vi "CalculateErrorInLeftPosition__slk_mt.vi"(3 "add error configure":T2, 7 "position in":T1, 8 "error in (no error)":errorcluster, 11 "origin (0,0)":T3) -> (0 "error out":errorcluster, 5 "position out":T1)   [LabVIEW 2012, in "Lazyboots Menu Tool.lvlib"]
doc: "Gets error in left position."
uses:
  Library/Lazyboots Menu Tool.lvlib
  <vilib>/Utility/miscctls.llb/LVPointTypeDef.ctl
  TypeDef/TypeDef_AddErrorConfigure__slk_mt.ctl
  <vilib>/Utility/miscctls.llb/LVPositionTypeDef.ctl
panel:
  # "CalculateErrorInLeftPosition__slk_mt.vi\nGets error in left position.\n\nNOTICE -- YOU MUST LEAVE THIS NOTICE IN PLACE.\n\nCopyright (c) 2011, LIANG LIU Shawn.Liu.cn@gmail.com\nAll rights reserved.\n\nRedistribution and use in source and binary forms, with or without modification, are permitted provided that the following conditions are met:\n-Redistributions of source code must retain the above copyright notice, this list of conditions and the following disclaimer.\n-Redistributions in binary form must reproduce the above copyright notice, this list of conditions and the following disclaimer in the documentation and/or other materials provided with the distribution.\n-Neither the name of the eLp nor the names of its contributors may be used to endorse or promote products derived from this software without specific prior written permission.\n\nTHIS SOFTWARE IS PROVIDED BY THE COPYRIGHT HOLDERS AND CONTRIBUTORS \"AS IS\" AND ANY EXPRESS OR IMPLIED WARRANTIES, INCLUDING, BUT NOT LIMITED TO, THE IMPLIED WARRANTIES OF MERCHANTABILITY AND FITNESS FOR A PARTICULAR PURPOSE ARE DISCLAIMED. IN NO EVENT SHALL THE COPYRIGHT HOLDER OR CONTRIBUTORS BE LIABLE FOR ANY DIRECT, INDIRECT, INCIDENTAL, SPECIAL, EXEMPLARY, OR CONSEQUENTIAL DAMAGES (INCLUDING, BUT NOT LIMITED TO, PROCUREMENT OF SUBSTITUTE GOODS OR SERVICES; LOSS OF USE, DATA, OR PROFITS; OR BUSINESS INTERRUPTION) HOWEVER CAUSED AND ON ANY THEORY OF LIABILITY, WHETHER IN CONTRACT, STRICT LIABILITY, OR TORT (INCLUDING NEGLIGENCE OR OTHERWISE) ARISING IN ANY WAY OUT OF THE USE OF THIS SOFTWARE, EVEN IF ADVISED OF THE POSSIBILITY OF SUCH DAMAGE."
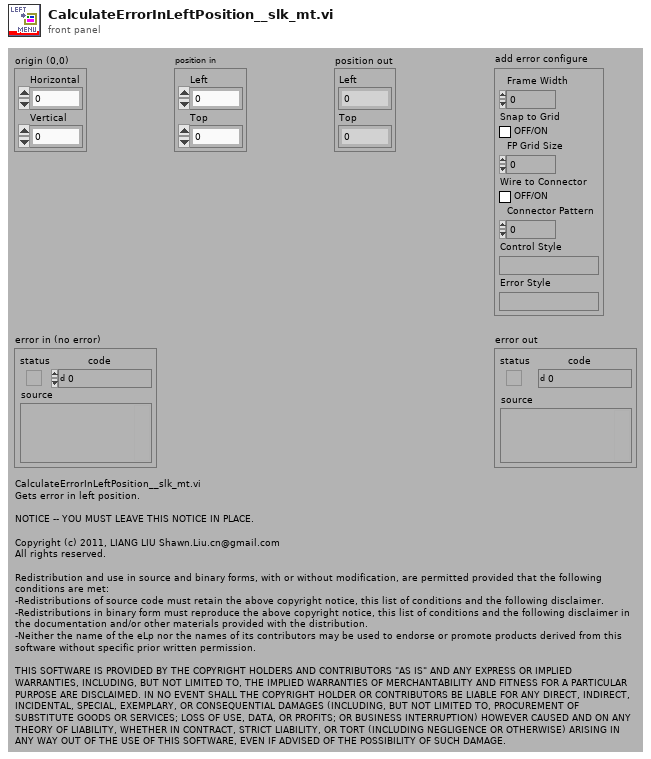
[diagram p1: front panel]
types:
  T1 = typedef "LVPositionTypeDef.ctl" = cluster{"Left":i32, "Top":i32}
  T2 = typedef "Lazyboots Menu Tool.lvlib/TypeDef_AddErrorConfigure__slk_mt.ctl" = cluster{"Frame Width":u32, "Snap to Grid":bool, "FP Grid Size":u32, "Wire to Connector":bool, "Connector Pattern":u32, "Control Style":string, "Error Style":string}
  T3 = typedef "LVPointTypeDef.ctl" = cluster{"Horizontal":i16, "Vertical":i16}
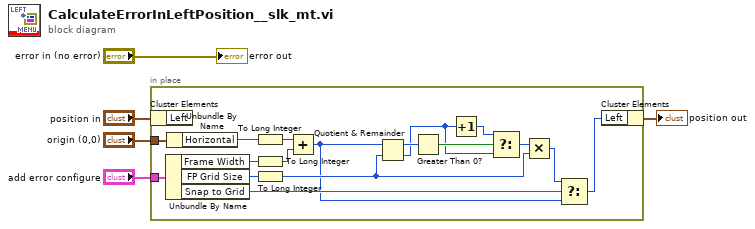
[diagram p0: block diagram]
diagram:
  n1 = in-place {
    in-place-border: "add error configure" -> [w12]
    in-place-border: "origin (0,0)" -> [w9]
    n2 = in-place-cluster #1("position in") -> ()  [unwired: 1 out]
    n3 = Unbundle By Name(w12) -> ("Frame Width"=w22:u32, "FP Grid Size"=w19:u32, "Snap to Grid"=w10:bool)
    n4 = Unbundle By Name(w9) -> ("Horizontal"=w21:i16)
    n5 = To Long Integer(number=w21) -> (32bit integer=w7:i32)
    n6 = To Long Integer(number=w22) -> (32bit integer=w20:i32)
    n7 = To Long Integer(number=w19) -> (32bit integer=w13:i32)
    n8 = Add(x=w7, y=w20) -> (x+y=w6:i32)
    n9 = Quotient & Remainder(x=w6, y=w13) -> (x-y*floor(x/y)=w15:i32, floor(x/y)=w14:i32)
    n10 = Greater Than 0?(x=w15) -> (x > 0?=w18:bool)
    n11 = Increment(x=w14) -> (x+1=w17:i32)
    n12 = Select(t=w17, s=w18, f=w14) -> (s? t:f=w16:i32)
    n13 = Multiply(x=w16, y=w13) -> (x*y=w11:i32)
    n14 = Select(t=w11, s=w10, f=w6) -> (s? t:f=w8:i32)
    n15 = in-place-cluster #1("Left"=w8) -> (→"position out":T1)
  }
  "error out" <- "error in (no error)"
